vi "AlliGator Convert FLI Dataset Info to String.vi"(5 "File Path":path, 8 "error in (no error)":errorcluster, 9 "size":i64, 10 "Metadata":string, 11 "FLI Parameters":T1) -> (0 "Error Out":errorcluster, 3 "Data Description":string)   [LabVIEW 2021, in "AlliGator HDF5.lvlib"]
doc: "Builds HDF5 Dataset Information string"
uses:
  AlliGator HDF5.lvlib
  Phasor/Phasor Fluorescence Lifetime Parameters v3.ctl
  Variant/Variant.lvlib
  Phasor/Phasor.lvlib
panel:
  # "see the AlliGator License on the block diagram (Ctrl+E or Window:Show Block Diagram)"
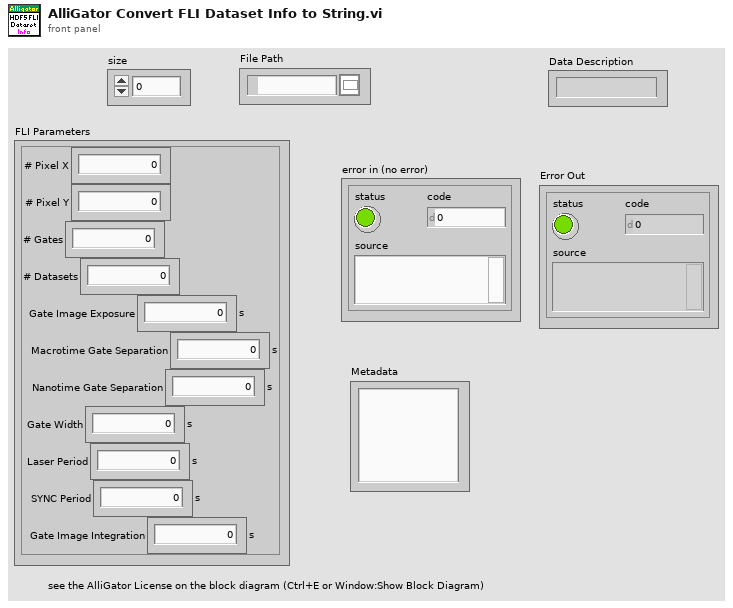
[diagram p1: front panel]
types:
  T1 = typedef "Phasor.lvlib/Phasor Fluorescence Lifetime Parameters v3.ctl" = cluster{"# Pixel X":i32, "# Pixel Y":i32, "# Gates":i32, "# Datasets":i32, "Gate Image Exposure":dbl[unit], "Macrotime Gate Separation":dbl[unit], "Nanotime Gate Separation":dbl[unit], "Gate Width":dbl[unit], "Laser Period":dbl[unit], "SYNC Period":dbl[unit], "Gate Image Integration":dbl[unit]}
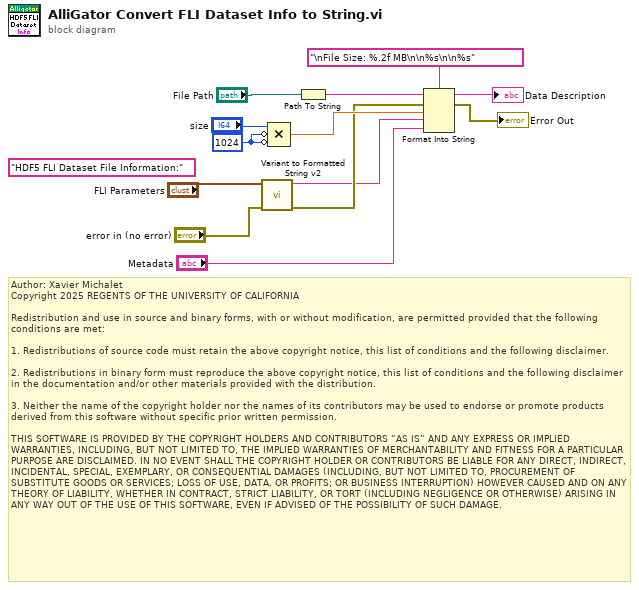
[diagram p0: block diagram]
diagram:
  w7 = i64 1024 ("y")
  (unwired) "HDF5 FLI Dataset File Information:" ("Label")
  # "Author: Xavier Michalet\nCopyright 2025 REGENTS OF THE UNIVERSITY OF CALIFORNIA\n\nRedistribution and use in source and binary forms, with or without modification, are permitted provided that the following conditions are met:\n\n1. Redistributions of source code must retain the above copyright notice, this list of conditions and the following disclaimer.\n\n2. Redistributions in binary form must reproduce the above copyright notice, this list of conditions and the following disclaimer in the documentation and/or other materials provided with the distribution.\n\n3. Neither the name of the copyright holder nor the names of its contributors may be used to endorse or promote products derived from this software without specific prior written permission.\n\nTHIS SOFTWARE IS PROVIDED BY THE COPYRIGHT HOLDERS AND CONTRIBUTORS “AS IS” AND ANY EXPRESS OR IMPLIED WARRANTIES, INCLUDING, BUT NOT LIMITED TO, THE IMPLIED WARRANTIES OF MERCHANTABILITY AND FITNESS FOR A PARTICULAR PURPOSE ARE DISCLAIMED. IN NO EVENT SHALL THE COPYRIGHT HOLDER OR CONTRIBUTORS BE LIABLE FOR ANY DIRECT, INDIRECT, INCIDENTAL, SPECIAL, EXEMPLARY, OR CONSEQUENTIAL DAMAGES (INCLUDING, BUT NOT LIMITED TO, PROCUREMENT OF SUBSTITUTE GOODS OR SERVICES; LOSS OF USE, DATA, OR PROFITS; OR BUSINESS INTERRUPTION) HOWEVER CAUSED AND ON ANY THEORY OF LIABILITY, WHETHER IN CONTRACT, STRICT LIABILITY, OR TORT (INCLUDING NEGLIGENCE OR OTHERWISE) ARISING IN ANY WAY OUT OF THE USE OF THIS SOFTWARE, EVEN IF ADVISED OF THE POSSIBILITY OF SUCH DAMAGE."
  n1 = call "Variant to Formatted String v2.vi"("error in (no error)"="error in (no error)", "Anything"="FLI Parameters") -> ("error out"=w5:errorcluster, "String"=w2:string)  [unwired: 8 in]
  n2 = Compound Arithmetic op=MULTIPLY("size", invert w7, invert w7) -> (w6:dbl)
  n3 = Path To String(path="File Path") -> (string=w10:string)
  n4 = Format Into String(format string="\nFile Size: %.2f MB\n\n%s\n\n%s", initial string=w10, error in=w5, w6, w2, "Metadata") -> (resulting string=→"Data Description":string, error out=→"Error Out":errorcluster)
